vi "Задание_АБ_новые_наработки.vi"() -> ()   [LabVIEW 2013]
uses:
  <vilib>/Analysis/NI_AALBase.lvlib
  <vilib>/gmath/NI_Gmath.lvlib
  <vilib>/Analysis/3filter.llb/Bessel Filter (DBL).vi
  <vilib>/gmath/statdist.llb/Beta Random.vi
  <vilib>/Analysis/baseanly.llb/Mean (DBL).vi
panel:
  out "Исходное сообщение":dbl[](array[numeric])
  out "Подготовленный к отправке мажоритарный код":dbl[][](array[numeric])
  out "2-х массив на выходе 3":dbl[][](array[numeric])
  in  "Размер окна":i32=4
  in  "Кол-во копий":i32=5
  out "Шум на основе распределения Рэлея":dbl[](graph)
  out "Итого. кол-во бит":i32
  in  "Пороговое значение":dbl
  out "Демодулированный и отфильтрованный сигнал":dbl[][](graph)
  out "Демодулированный сигнал":i16[](graph)
  in  "Нижняя частота среза":dbl
  in  "Порядок фильтра":i64(slide) scale=0.0..20.0
  in  "Переменная floor(x/y)":i32
  out "Модулирующий сигнал":dbl[](graph)
  out "Частотно модулированный цифровой сигнал":dbl[](graph)
  in  "см. 1.2 Циклов в секунду":i32(slide) scale=4.0..50.0
  in  "Сколько битов брать":i32=4
  out "Радио сигнал с паузами":dbl[](graph)
  in  "Кол-во выборок":i32=400
  out "Массив с паузами":dbl[](array[numeric])
  in  "Количество бит":i32=8
  out "Вырезка из массива":dbl[](array[numeric])
  out "Биты на выходе 1":dbl[](array[numeric])
  # "Демодуляция"
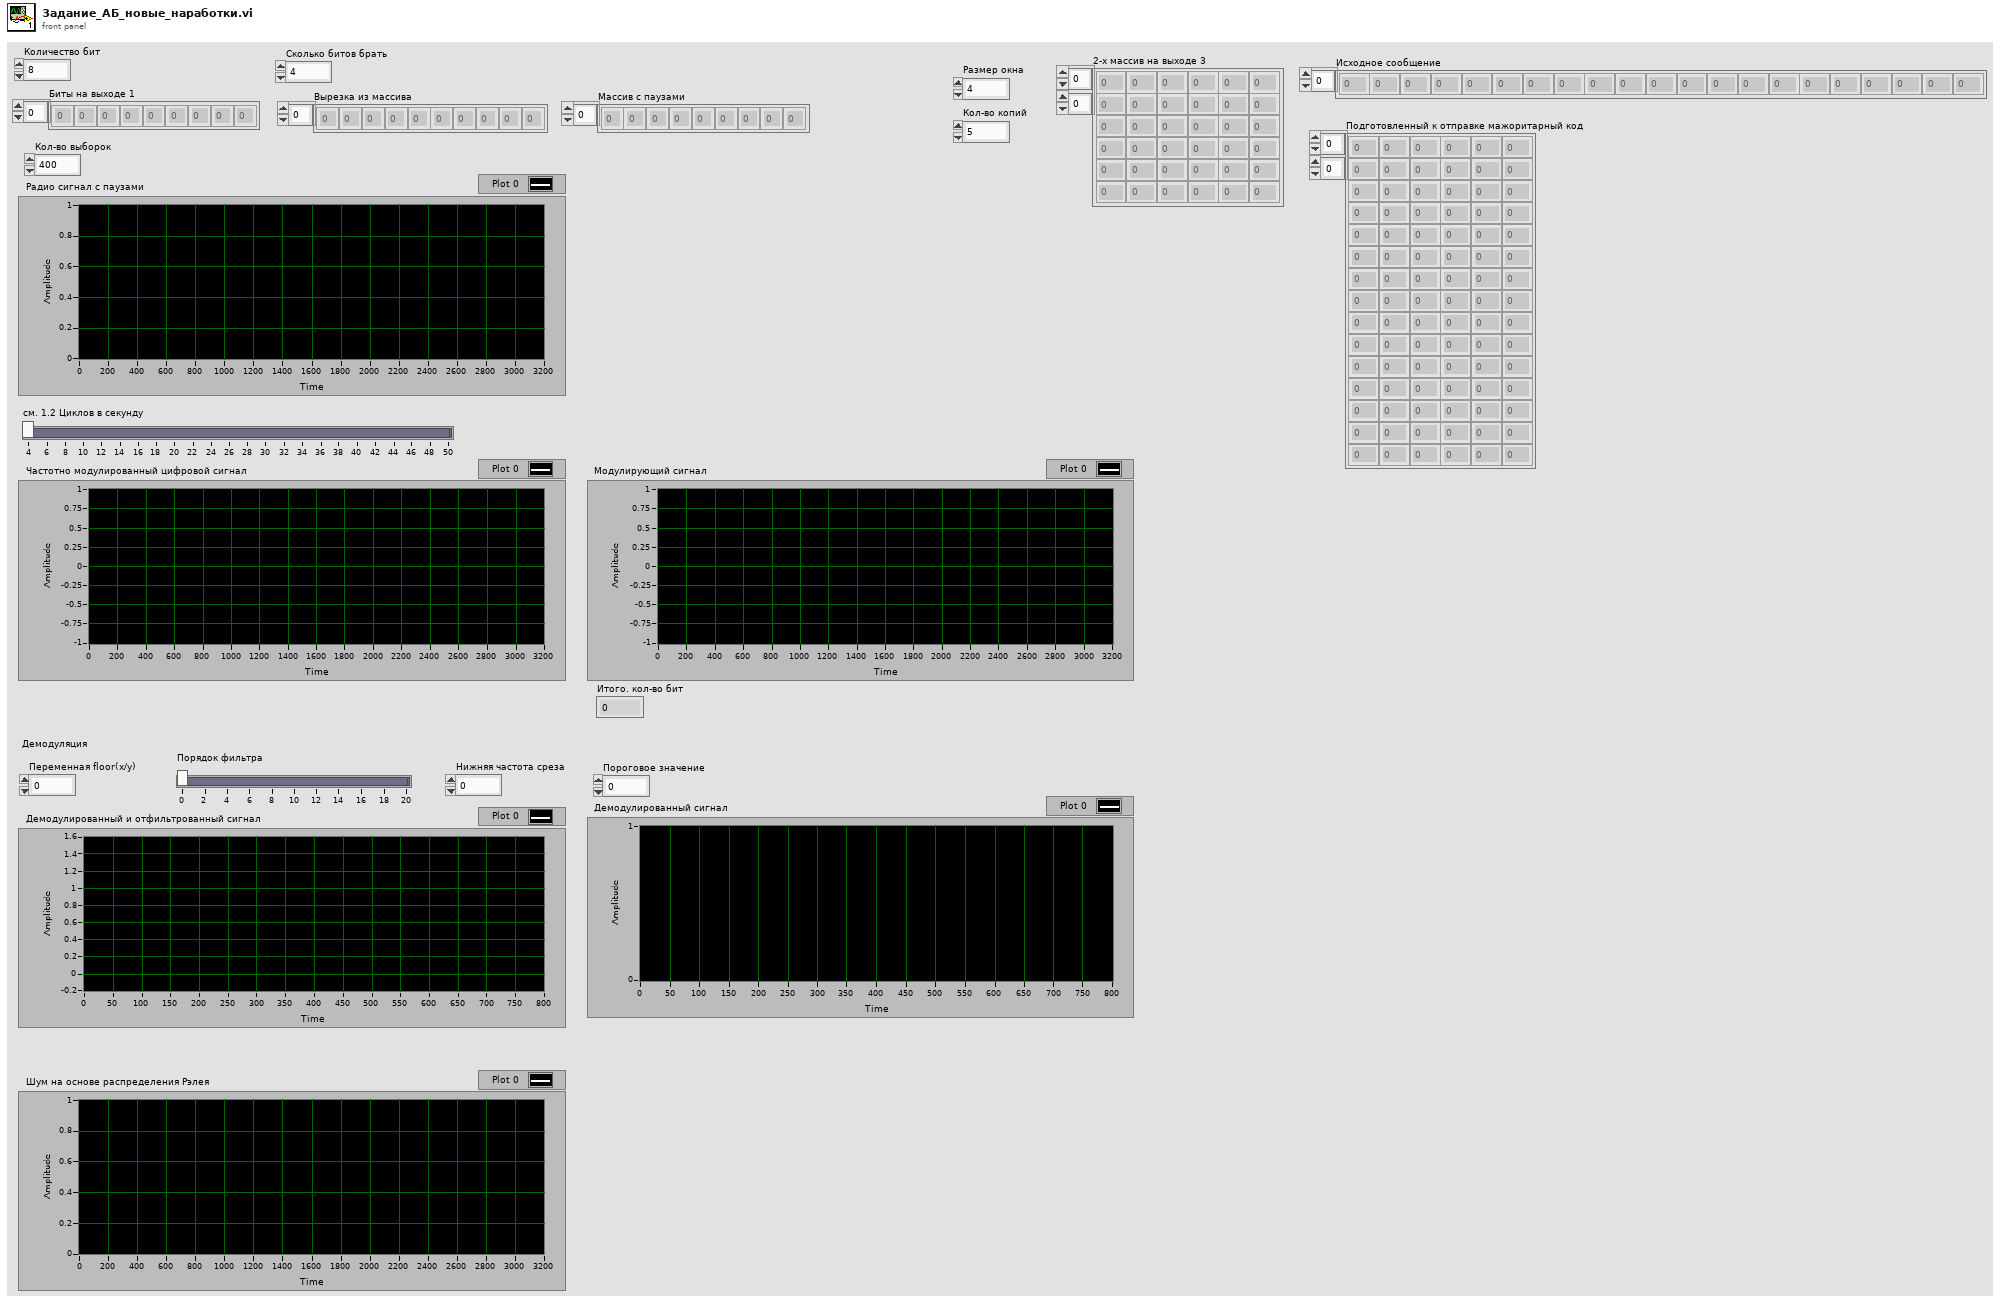
[diagram p1: front panel]
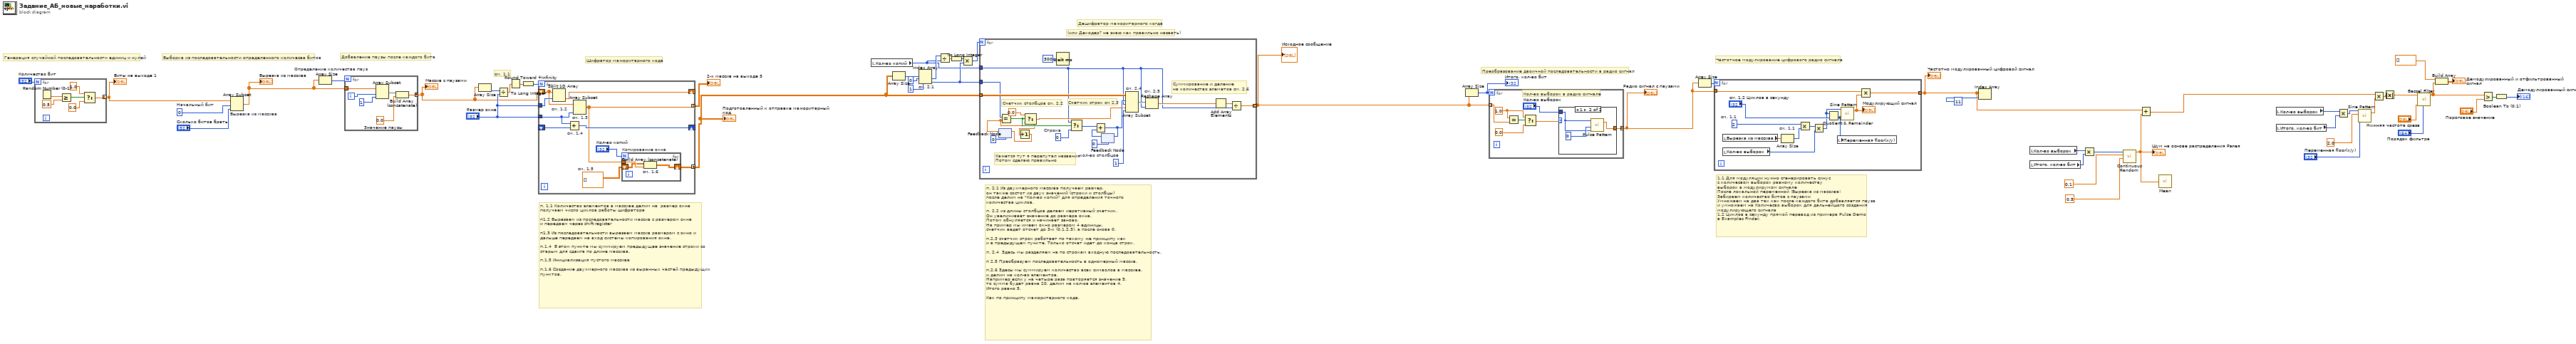
[diagram p0: block diagram]
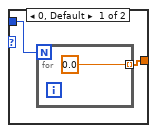
[diagram p2: hidden frame]
diagram:
  w51 = 0  # Начальный бит
  # "п. 2.1 Из двухмерного массива получаем размер.\nон также состот из двух значений (строки и столбцы) \nпосле делим на \"Кол-во копий\" для определения точного\nколичества циклов.\n\nп. 2.2 из длины столбцов делаем иеративный счетчик. \nОн увеличивает значение до размера окна.\nПотом обнуляется и начинает заново.\nНа пример мы имеем окно размером 4 единицы.\nсчетчик ведет отсчет до 3-х (0,1,2,3), а после снова 0.\n\nп.2.3 счетчик строк работает по такому же принципу как \nи в предыдущем пункте. Только отсчет идет до конца строк.\n\nп. 2.4  Здесь мы разделяем на по строкам входную последовательность.\n\nп 2.5 Преобразуем последовательность в одномерный массив.\n\nп.2.6 Здесы мы суммируем количество всех символов в массиве.\nи делим на кол-во элементов.\nНапример если у на четыре раза повторяется значение 5, \nто сумма будет равна 20, делим на кол-ов элементов 4. \nИтого равно 5. \n\nКак по принципу мажоритарного кода."
  # "см. 1.1"
  # "(или Декодер? не знаю как правильно назвать)"
  # "Дешифратор мажоритарного когда"
  # "п. 1.1 Количество элементов в массиве делим на  размер окна\nполучаем число циклов работы шифратора\n\nп1.2 Вырезаем из последовательности массив с размером окна \nи передаем через shift register\n\nп1.3 Из последовательности вырезаем массив размером с окно и \nдальше передаем на вход системы копирования окна.\n \nп.1.4  В этом пункте мы суммируем предыдущее значение строки со\nстарым для сдвига по длине массива.\n\nп.1.5 Инициализация пустого массива\n\nп.1.6 Создание двухмерного массива из выранных частей предыдущих\nпунктов."
  # "Шифратор мажоритарного кода"
  # "1.1 Для модуляции нужно сгенерировать синус \nс количесвом выборок равному количеству \nвыборок в модулирумом сигнале\nПосле локальной переменной !Вырезка из массива! \nЗабираем количество битов с паузами \nУмножаем на два так как после каждого бита добавляется пауза\nи умножаем на Количесво выборок для дальнейшого создания  \nмодулирующего сигнала\n1.2 Циклов в секунду прямой перевод из примера Pulse Demo \nв Examples Finder."
  # "Преобразование двоичной последовательности в радио сигнал"
  # "Частотное модулирование цифрового радио сигнала"
  # "Добавление паузы после каждого бита"
  # "Выборка из последовательности определенного количесва битов"
  # "Генерация случайной последовательности единиц и нулей"
  n1 = for {
    N: "Количество бит" -> [_]
    tunnel: [w53] -> w49 mode=indexing
    n2 = Random Number (0-1)() -> (number: 0 to 1=w58:dbl)
    n3 = Greater Or Equal?(x=w58, y=0.5) -> (x >= y?=w56:bool)
    n4 = Select(t=1.0, s=w56, f=0.0) -> (s? t:f=w53:dbl)
  }
  "Биты на выходе 1" <- w49
  n5 = Array Subset "Вырезка из массива"(array=w49, index=w51, length="Сколько битов брать") -> (w47:dbl[])
  "Вырезка из массива" <- w47
  n6 = Array Size "Определение количества пауз"(array=w47) -> (size(s)=w48:i32)
  n7 = for {
    N: w48 -> [_]
    tunnel: w47 -> [w61]
    tunnel: [w60] -> w12 mode=concatenating
    i -> [w59]
    w62 = 0.0  # Значение паузы
    n8 = Array Subset(array=w61, index=w59, length=1) -> (w63:dbl[])
    n9 = Build Array (concatenate)(w63, w62) -> (w60:dbl[])
  }
  "Массив с паузами" <- w12
  n10 = Array Size(array=w12) -> (size(s)=w18:i32)
  n11 = Divide(x=w18, y="Размер окна") -> (x/y=w17:dbl)
  n12 = Round Toward +Infinity(x=w17) -> (ceil(x): smallest int >= x=w16:dbl)
  n13 = To Long Integer(number=w16) -> (32bit integer=w13:i32)
  n14 = for {
    N: w13 -> [_]
    shift-right: [w74] -> _
    shift-left: w12 -> [w72]
    tunnel: "Размер окна" -> [w73]
    shift-right: [w70] -> _
    shift-left: _ -> [w69]
    tunnel: "Размер окна" -> [w71]
    tunnel: [w67] -> w14 mode=indexing
    tunnel: [w66] -> w1 mode=concatenating
    w65 = dbl[][] []  # см. 1.5
    n15 = Split 1D Array "см. 1.2"(array=w72, index=w73) -> (second subarray=w74:dbl[])  [unwired: 1 out]
    n16 = Add "см. 1.4"(x=w71, y=w69) -> (x+y=w70:i32)
    n17 = Array Subset "см. 1.3"(array=w72, length=w71) -> (w67:dbl[])  [unwired: 1 in]
    n18 = for "Копирование окна" {
      N: "Кол-во копий" -> [_]
      tunnel: w67 -> [w76]
      shift-right: [w77] -> w66
      shift-left: w65 -> [w75]
      n19 = Build Array (concatenate) "см. 1.6"(w75, w76) -> (w77:dbl[][])
    }
  }
  "2-х массив на выходе 3" <- w14
  "Подготовленный к отправке мажоритарный код" <- w1
  n20 = local read "Кол-во копий"() -> (w3:i32)
  n21 = Array Size(array=w1) -> (size(s)=w11:i32[])
  n22 = Index Array "см. 2.1"(array=w11, index #1=0 ("index"), index #2=1 ("index")) -> (element #1=w8:i32, element #2=w7:i32)
  n23 = Divide(x=w8, y=w3) -> (x/y=w6:dbl)
  n24 = To Long Integer(number=w6) -> (32bit integer=w5:i32)
  n25 = Multiply(x=w5, y=w7) -> (x*y=w4:i32)
  n26 = for {
    N: w4 -> [_]
    tunnel: w1 -> [w96]
    tunnel: w7 -> [w88]
    tunnel: w3 -> [w79]
    tunnel: [w78] -> w2 mode=indexing
    w95 = 1  # кол-во столбцов
    w86 = 0  # Строка
    # "Суммирование и деление \nна количество элеметов см. 2.6"
    # "Кажется тут я перепутал названия  \nПотом сделаю правильно"
    # "Счетчик строк см 2.3"
    # "Счетчик столбцов см. 2.2"
    n27 = feedback #1(0) -> (w84:dbl)
    n28 = Equal?(x=w88, y=w84) -> (x = y?=w90:bool)
    n29 = Select(t=0.0, s=w90, f=w84) -> (s? t:f=w83:dbl)
    n30 = Increment(x=w83) -> (x+1=w82:dbl)
    n31 = feedback-in #1(w82) -> ()
    n32 = Wait (ms)(milliseconds to wait=u32 300) -> ()  [unwired: 1 out]
    n33 = Select(t=w79, s=w90, f=w86) -> (s? t:f=w87:i32)
    n34 = feedback #2(0) -> (w89:i32)
    n35 = Add(x=w87, y=w89) -> (x+y=w85:i32)
    n36 = feedback-in #2(w85) -> ()
    n37 = Array Subset "см. 2.4"(array=w96, index (row)=w85, length (row)=w79, index (col)=w83, length (col)=w95) -> (w97:dbl[][])
    n38 = Reshape Array "см. 2.5"(w97, w79) -> (w81:dbl[])
    n39 = Add Array Elements(numeric array=w81) -> (sum=w80:dbl)
    n40 = Divide(x=w80, y=w79) -> (x/y=w78:dbl)
  }
  "Исходное сообщение" <- w2
  n41 = Array Size(array=w2) -> (size(s)=w45:i32)
  "Итого. кол-во бит" <- w45
  n42 = for {
    N: w45 -> [_]
    tunnel: w2 -> [w101] mode=indexing
    tunnel: [w99] -> w44 mode=concatenating
    w103 = 1.0
    # "Кол-во выборок в радио сигнале"
    n43 = Equal?(x=w103, y=w101) -> (x = y?=w104:bool)
    n44 = Select(t=w103, s=w104, f=0.0) -> (s? t:f=w100:dbl)
    n45 = case shown="1" w100 {
      tunnel: [w105 w109] -> w99
      tunnel: "Кол-во выборок" -> [w106 w108]
      frame 0, Default {
        n46 = for {
          N: w106 -> [_]
          tunnel: [0.0] -> w105 mode=indexing
        }
      }
      frame 1 {
        n47 = call <vilib>:"Pulse Pattern.vi"("width"=w108, "delay"=0, "samples"=w108) -> ("Pulse Pattern"=w109:dbl[])  [unwired: 1 in, 1 out]
      }
    }
  }
  "Радио сигнал с паузами" <- w44
  n48 = Array Size(array=w44) -> (size(s)=w46:i32)
  n49 = for {
    N: w46 -> [_]
    tunnel: w44 -> [w120]
    tunnel: [w119] -> w20
    w115 = 2  # см. 1.1
    n50 = local read "Вырезка из массива"() -> (w117:dbl[])
    n51 = local read "Кол-во выборок"() -> (w113:i32)
    n52 = Array Size "см. 1.1"(array=w117) -> (size(s)=w116:i32)
    n53 = Multiply(x=w115, y=w116) -> (x*y=w114:i32)
    n54 = Multiply(x=w114, y=w113) -> (x*y=w112:i32)
    n55 = Quotient & Remainder(x=w112, y="см. 1.2 Циклов в секунду") -> (floor(x/y)=w111:i32)  [unwired: 1 out]
    n56 = local write "Переменная floor(x/y)"(w111) -> ()
    n57 = call <vilib>:"Sine Pattern.vi"("cycles"=w111, "samples"=w112) -> ("Sinusoidal Pattern"=w118:dbl[])  [unwired: 2 in, 1 out]
    "Модулирующий сигнал" <- w118
    n58 = Multiply(x=w120, y=w118) -> (x*y=w119:dbl[])
  }
  "Частотно модулированный цифровой сигнал" <- w20
  n59 = Index Array(array=w20, index=11 ("index (row)")) -> ()  [unwired: 1 out]
  n60 = local read "Кол-во выборок"() -> (w24:i32)
  n61 = local read "Итого. кол-во бит"() -> (w23:i32)
  n62 = Multiply(x=w24, y=w23) -> (x*y=w22:i32)
  n63 = call-poly <vilib>:"Continuous Random.vi"("b"=0.5, "a"=0.1 ("x"), "samples"=w22) -> ("beta random data"=w21:dbl[])  [unwired: 7 in, 1 out]
  "Шум на основе распределения Рэлея" <- w21
  n64 = Add(x=w20, y=w21) -> (x+y=w19:dbl[])
  n65 = call-poly <vilib>:"Mean.vi"("X"=w21) -> ()  [unwired: 2 out]
  n66 = local read "Кол-во выборок"() -> (w28:i32)
  n67 = local read "Итого. кол-во бит"() -> (w27:i32)
  n68 = Multiply(x=w28, y=w27) -> (x*y=w29:i32)
  n69 = call <vilib>:"Sine Pattern.vi"("cycles"="Переменная floor(x/y)", "amplitude"=2.0, "samples"=w29) -> ("Sinusoidal Pattern"=w31:dbl[])  [unwired: 1 in, 1 out]
  n70 = Multiply(x=w19, y=w31) -> (x*y=w40:dbl[])
  n71 = Absolute Value(x=w40) -> (abs(x)=w37:dbl[])
  n72 = call-poly <vilib>:"Bessel Filter.vi"("order"="Порядок фильтра", "low cutoff freq: fl"="Нижняя частота среза", "X"=w37) -> ("Filtered X"=w35:dbl[])  [unwired: 5 in, 1 out]
  n73 = Build Array(dbl[] [] ("element"), w35) -> (→"Демодулированный и отфильтрованный сигнал":dbl[][])
  n74 = Greater?(x=w35, y="Пороговое значение") -> (0:w34:bool[])
  n75 = Boolean To (0,1)(Boolean=w34) -> (0, 1=→"Демодулированный сигнал":i16[])
